vi "Load and Save Data (FIR Data).vi"(0 "VISA resource name":refnum<visa-resource-name>, 1 "FIR Coefficients":dbl[](array[numeric])=[0.0, 0.0], 5 "Destination File":string, 7 "Filter Type (0: Real)":u16(ring) items=["Real", "Complex"], 9 "OSR(1)":i32=1, 11 "error in (no error)":errorcluster) -> (4 "VISA resource name out":refnum<visa-resource-name>, 15 "error out":errorcluster)   [LabVIEW 2018, in "Agilent PSG MXG Series.lvlib"]
doc: "Loads user-defined finite impulse response (FIR) coefficient data, with a given oversample ratio (OSR), into a file in the signal generator's non-volatile memory. \n\n<B>Notes:</B>\n(1) This VI is valid in N5172B that installs with <B>Option 653</B> or <B>Option 655</B>, or N5182B that installs with <B>Option 656</B> or <B>Option 657</B>.\n(2) This VI is valid in N5162A/82A that installs with <B>Option 651</B>, <B>Option 652</B>, or <B>Option 654</B>."
uses:
  Agilent PSG MXG Series.lvlib
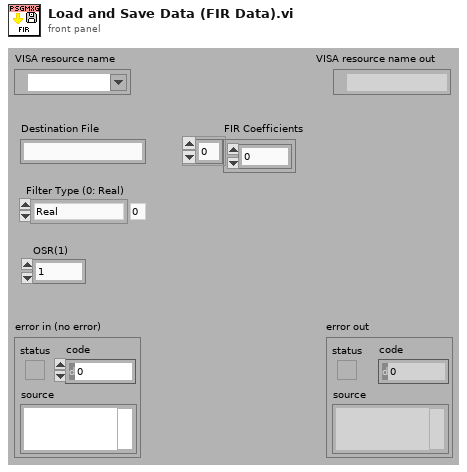
[diagram p1: front panel]
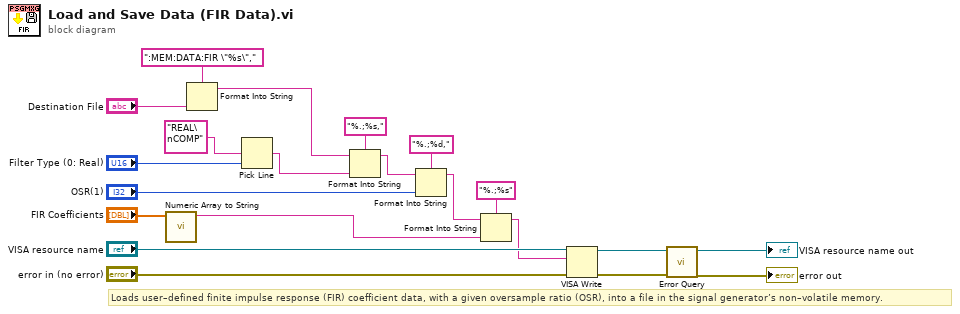
[diagram p0: block diagram]
diagram:
  # "Loads user–defined finite impulse response (FIR) coefficient data, with a given oversample ratio (OSR), into a file in the signal generator’s non–volatile memory."
  n1 = call "Numeric Array to String.vi"("Numeric Array"="FIR Coefficients") -> ("Output String"=w3:string)  [unwired: 10 in]
  n2 = Format Into String(format string=":MEM:DATA:FIR \"%s\",", "Destination File") -> (resulting string=w11:string)  [unwired: 2 in, 1 out]
  n3 = Pick Line(multi-line string="REAL\nCOMP", line index="Filter Type (0: Real)") -> (output string=w10:string)  [unwired: 1 in]
  n4 = Format Into String(format string="%.;%s,", initial string=w11, w10) -> (resulting string=w8:string)  [unwired: 1 in, 1 out]
  n5 = Format Into String(format string="%.;%d,", initial string=w8, "OSR(1)") -> (resulting string=w4:string)  [unwired: 1 in, 1 out]
  n6 = Format Into String(format string="%.;%s", initial string=w4, w3) -> (resulting string=w2:string)  [unwired: 1 in, 1 out]
  n7 = VISA Write(VISA resource name="VISA resource name", write buffer=w2, error in (no error)="error in (no error)") -> (VISA resource name out=w21:refnum<visa-resource-name>, error out=w20:errorcluster)  [unwired: 1 out]
  n8 = call "Error Query.vi"("error in (no error)"=w20, "VISA resource name"=w21) -> ("error out"=→"error out":errorcluster, "VISA resource name out"=→"VISA resource name out":refnum<visa-resource-name>)  [unwired: 6 in, 2 out]
